vi "Write Page Selector Visible.vi"(8 "error in (no error)":errorcluster, 10 "PageSelVis":bool, 11 "PageSelector.lvclass in":refnum<class "PageSelector.lvclass">) -> (0 "error out":errorcluster, 3 "PageSelector.lvclass out":refnum<class "PageSelector.lvclass">)   [LabVIEW 2015, in "PageSelector.lvclass"]
uses:
  PageSelector.lvclass
  PageSelector.lvclass/PageSelector.ctl
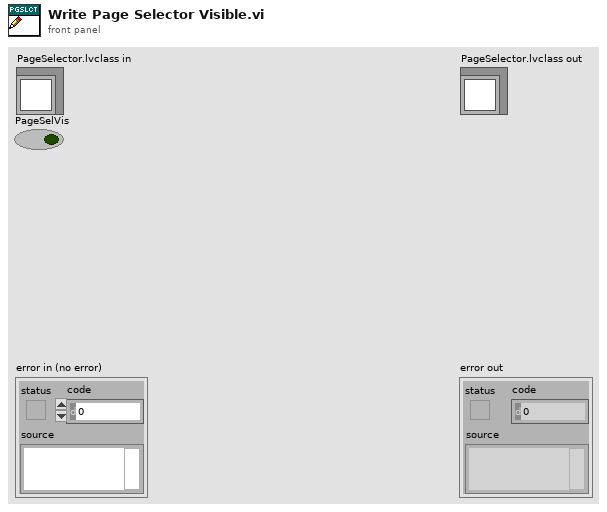
[diagram p1: front panel]
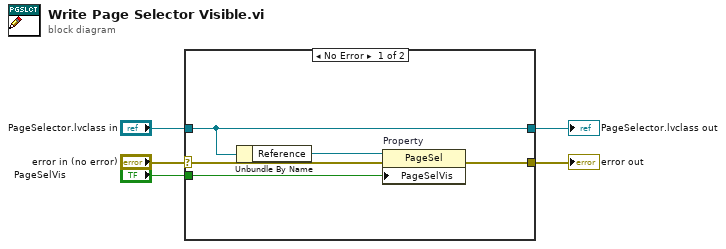
[diagram p0: block diagram]
diagram:
  n1 = case shown="No Error" "error in (no error)" {
    selector: "error in (no error)" -> [w6 w12]
    tunnel: [w10 w12] -> w4
    tunnel: [w8 w11] -> w2
    tunnel: "PageSelector.lvclass in" -> [w8 w11]
    tunnel: "PageSelVis" -> [w9 _]
    frame No Error {
      n2 = Unbundle By Name(w8) -> ("Reference"=w7:refnum<vi>)
      n3 = property on="Property" class="PageSel"(reference=w7, error in=w6, "PageSelVis"=w9) -> (error out=w10:errorcluster)  [unwired: 1 out]
    }
    frame Error {
    }
  }
  "error out" <- w4
  "PageSelector.lvclass out" <- w2
